vi "niTuner Set Freq(f array).vi"(8 "error in":errorcluster, 9 "spans":dbl[](array[numeric]) format="%.2f", 10 "desired RF frequencies":dbl[](array[numeric]) format="%.2f", 11 "taskID in":i32 format="%.0x") -> (0 "error out":errorcluster, 1 "actual RF tuned frequencies":dbl[](array[numeric]) format="%.2f", 2 "actual IF frequencies":dbl[](array[numeric]) format="%.2f", 3 "taskID out":i32 format="%.0x", 4 "frequency shifts":dbl[](array[numeric]) format="%.2f")   [LabVIEW 2011]
doc: "This polymorph sets multiple center frequencies (up to 720) in the scan list. The PXI-5600 downconverter will not advance to the first frequency until niTuner Initiate Scan.vi is called. When triggered, the PXI-5600 downconverter tunes to the scan list frequencies in succession. Each frequency is associated with a span.\n\nNOTE: If new center frequencies of less than 15 MHz are specified by a call to this VI, attenuation is automatically adjusted. This may add an additional 20 dB attenuation."
uses:
  nipxi5600u.dll
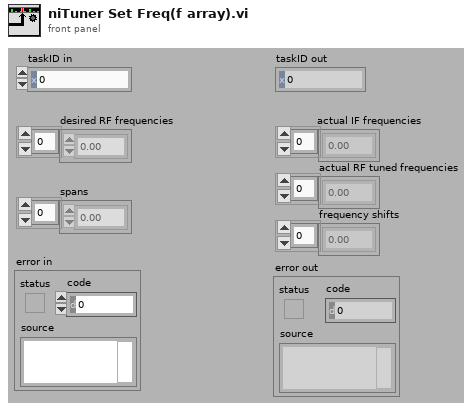
[diagram p1: front panel]
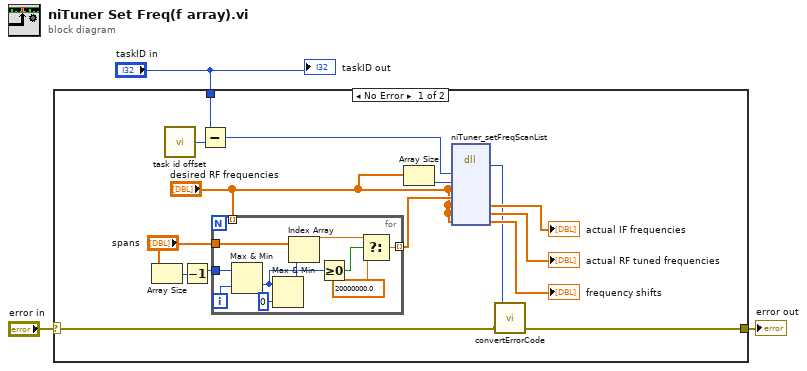
[diagram p0: block diagram]
diagram:
  n1 = case shown="No Error" "error in" {
    selector: "error in" -> [w13 w29]
    tunnel: [w12 w29] -> w2
    tunnel: "taskID in" -> [w4 _]
    frame No Error {
      n2 = Array Size(array="spans") -> (size(s)=w10:i32)
      n3 = call <instrlib>:"task id offset.vi"() -> ("taskID offset"=w5:i32)
      n4 = Decrement(x=w10) -> (x-1=w9:i32)
      n5 = Subtract(x=w4, y=w5) -> (x-y=w6:i32)
      n6 = for {
        tunnel: "desired RF frequencies" -> [_] mode=indexing
        tunnel: "spans" -> [w28]
        tunnel: w9 -> [w27]
        tunnel: [w22] -> w8 mode=indexing
        i -> [w26]
        n7 = Max & Min(x=w27, y=w26) -> (min(x,y)=w23:i32)  [unwired: 1 out]
        n8 = Max & Min(x=w23, y=0 ("lower limit")) -> (max(x,y)=w24:i32)  [unwired: 1 out]
        n9 = Index Array(array=w28, index=w24) -> (element=w20:dbl)
        n10 = Greater Or Equal To 0?(x=w23) -> (x >= 0?=w21:bool)
        n11 = Select(t=w20, s=w21, f=20000000.0) -> (s? t:f=w22:dbl)
      }
      n12 = Array Size(array="desired RF frequencies") -> (size(s)=w18:i32)
      n13 = dll-call lib="nipxi5600u.dll" fn="niTuner_setFreqScanList"("taskID"=w6, "listSize"=w18, "desiredRFcenterFrequencies"="desired RF frequencies", "spans"=w8, "actualIFcenterFrequency"="desired RF frequencies", "actualRFcenterFrequencies"="desired RF frequencies", "freqShifts"="desired RF frequencies") -> (w14:i32, "actualIFcenterFrequency"=→"actual IF frequencies":dbl[], "actualRFcenterFrequencies"=→"actual RF tuned frequencies":dbl[], "freqShifts"=→"frequency shifts":dbl[])  [unwired: 7 in, 2 out]
      n14 = call <instrlib>:"convertErrorCode.vi"("error in"=w13, "error code"=w14) -> ("error out"=w12:errorcluster)
    }
    frame Error {
    }
  }
  "error out" <- w2
  "taskID out" <- "taskID in"
